vi "NI9234SampleRates.vi"(11 "RequestedFrequency(Hz)":dbl) -> (3 "ClosestHigherFrequency(Hz)":dbl)   [LabVIEW 2015]
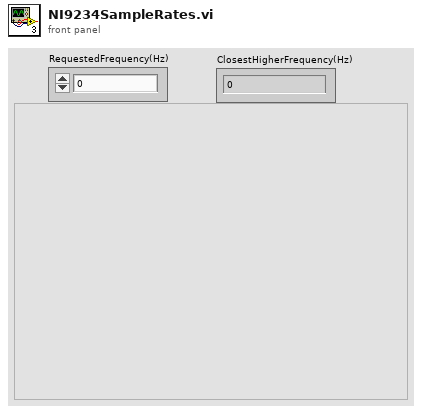
[diagram p1: front panel]
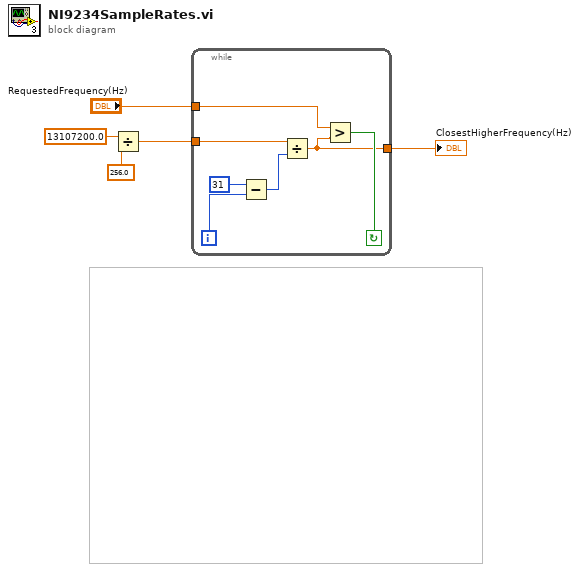
[diagram p0: block diagram]
diagram:
  n1 = Divide(x=13107200.0, y=256.0) -> (x/y=w3:dbl)
  n2 = while {
    tunnel: w3 -> [w10]
    tunnel: "RequestedFrequency(Hz)" -> [w8]
    tunnel: [w6] -> w1
    i -> [w12]
    stop <- w7 continue-if-true
    n3 = Subtract(x=31, y=w12) -> (x-y=w9:i32)
    n4 = Divide(x=w10, y=w9) -> (x/y=w6:dbl)
    n5 = Greater?(x=w8, y=w6) -> (0:w7:bool)
  }
  "ClosestHigherFrequency(Hz)" <- w1
